vi "Data Sharing Framework Configuration Explorer.vi"(6 "menu options":cluster{"open":bool, "save":bool, "view":bool}={"open"=TRUE, "save"=FALSE, "view"=FALSE}, 8 "error in (no error)":errorcluster, 11 "Path in":path) -> (0 "error out":errorcluster, 3 "Path out":path)   [LabVIEW 2017]
uses:
  Main VI/Application Data.ctl
  VeriStand/Data Sharing Custom Device/Source/DSF Core.lvlibp/DSF Configuration API/Configuration Session.lvclass
  Main VI/View Mode.ctl
  Main VI/Load DSF Configuration File.vi
  Item Tree/Clear Tree.vi
  VeriStand/Data Sharing Custom Device/Source/DSF Core.lvlibp/DSF Configuration API/Public/Read DSF Version.vi
  Value Tree/variant to tree resources/View Variant in Tree.vi
  VeriStand/Data Sharing Custom Device/Source/DSF Core.lvlibp/DSF Configuration API/Private/File IO/Read Configuration Version.vi
  Item Tree/Get Item Type.vi
  Item Tree/Get Item Display Name.vi
  VeriStand/Data Sharing Custom Device/Source/DSF Core.lvlibp/DSF Configuration API/Public/Read Item.vi
  VeriStand/Data Sharing Custom Device/Source/DSF Core.lvlibp/DSF Configuration API/Public/Read Item/Read Group.vi
  VeriStand/Data Sharing Custom Device/Source/DSF Core.lvlibp/DSF Configuration API/Public/Read Item/Read Transfer.vi
  VeriStand/Data Sharing Custom Device/Source/DSF Core.lvlibp/DSF Configuration API/Public/Read Item/Read Channel.vi
  VeriStand/Data Sharing Custom Device/Source/DSF Core.lvlibp/DSF Configuration API/Public/Read Item/Read Settings.vi
  VeriStand/Data Sharing Custom Device/Source/DSF Core.lvlibp/DSF Configuration API/Public/Read Item/Read Plugin.vi
  DSF Configuration Utility.lvlib
panel:
  in  "Item Tree":string(tree)
  in  "Value Tree":string(tree)
  # "DSF Configuration Explorer"
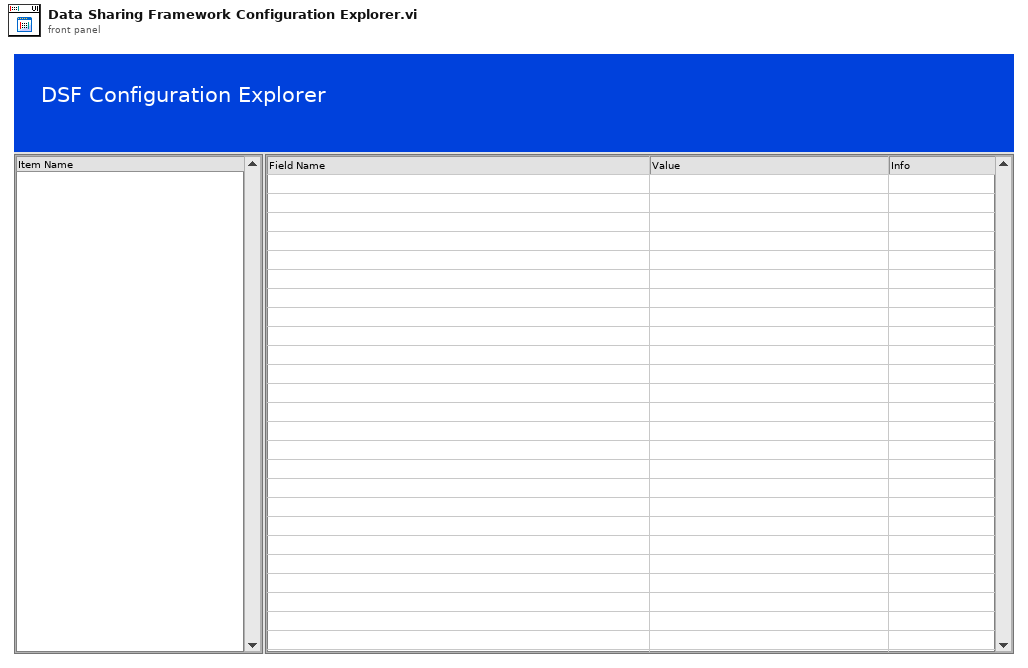
[diagram p1: front panel]
types:
  T1 = typedef "DSF Configuration Utility.lvlib/View Mode.ctl" = enum16{"Tree", "List"}
  T2 = typedef "DSF Configuration Utility.lvlib/Application Data.ctl" = cluster{"Item Tree Control":refnum<vi>, "Value Tree Control":refnum<vi>, "DSF Refnum":refnum<class "Configuration Session.lvclass">, "Top-Level VI":refnum<vi>, "View State":T1, "menu reference":refnum<k9>}
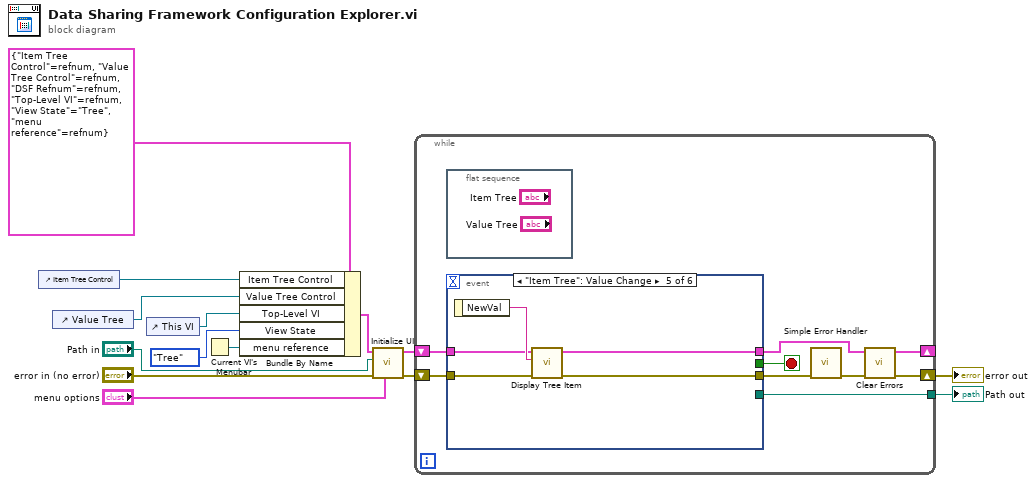
[diagram p0: block diagram]
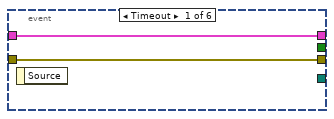
[diagram p2: hidden frame]
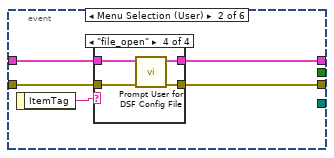
[diagram p3: hidden frame]
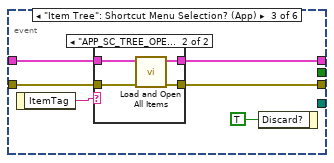
[diagram p7: hidden frame]
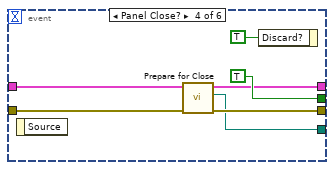
[diagram p9: hidden frame]
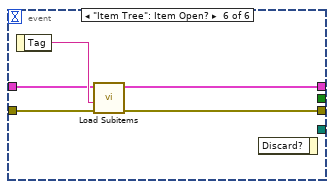
[diagram p10: hidden frame]
diagram:
  n1 = control-ref of="Item Tree Control"() -> (w2:refnum<vi>)
  n2 = control-ref of="Value Tree"() -> (w1:refnum<vi>)
  n3 = control-ref of="This VI"() -> (w11:refnum<vi>)
  n4 = Current VI's Menubar() -> (w6:refnum<k9>)
  n5 = Bundle By Name(cluster=T2 {"Item Tree Control"=refnum, "Value Tree Control"=refnum, "DSF Refnum"=refnum, "Top-Level VI"=refnum, "View State"=enum."Tree", "menu reference"=refnum}, "Item Tree Control"=w2, "Value Tree Control"=w1, "Top-Level VI"=w11, "View State"=View_Mode."Tree", "menu reference"=w6) -> (w4:T2)
  n6 = call "Initialize UI.vi"("menu options"="menu options", "error in (no error)"="error in (no error)", "Path"="Path in", "Application Data in"=w4) -> ("error out"=w14:errorcluster, "Application Data out"=w10:T2)  [unwired: 6 in]
  n7 = while {
    shift-right: [w15] -> w7
    shift-left: w14 -> [w21]
    shift-right: [w17] -> _
    shift-left: w10 -> [w18]
    tunnel: [w16] -> w8
    stop <- w22 stop-if-true
    n8 = flat-sequence {
      frame #0 {
      }
    }
    n9 = event shown="[4] \"Item Tree\": Value Change" {
      selector: _ -> [_ _ _ _ _ _]
      dyn-events: _ -> [_ _ _ _ _ _]
      timeout: _ -> [_ _ _ _ _ _]
      tunnel: [_ _ _ TRUE _ _] -> w22
      tunnel: w21 -> [w24 w28 w42 w57 w63 w68]
      tunnel: [w24 w27 w43 w54 w61 w67] -> w19
      tunnel: w18 -> [w23 w26 w44 w55 w59 w65]
      tunnel: [w23 w25 w40 w53 w60 w64] -> w17
      tunnel: [_ _ _ w52 _ _] -> w16
      event Timeout {
        n10 = event-data() -> ()  [unwired: 1 in, 1 out]
      }
      event Menu Selection (User) {
        n11 = event-data() -> ("ItemTag"=w29:string)  [unwired: 1 in]
        n12 = case shown="\"file_open\"" w29 {
          tunnel: [w30 w32 w34 w38] -> w25
          tunnel: [w31 w33 w35 w37] -> w27
          tunnel: w28 -> [w31 w33 w35 w39]
          tunnel: w26 -> [w30 w32 w34 w36]
          frame "view_tree" {
          }
          frame "view_list" {
          }
          frame Default {
          }
          frame "file_open" {
            n13 = call "Prompt User for DSF Config File.vi"("error in (no error)"=w39, "Application Data in"=w36) -> ("error out"=w37:errorcluster, "Application Data out"=w38:T2)  [unwired: 8 in]
          }
        }
      }
      event "Item Tree": Shortcut Menu Selection? (App) {
        n14 = event-data() -> ("ItemTag"=w45:string)  [unwired: 1 in]
        n15 = case shown="\"APP_SC_TREE_OPEN_ALL_ITEMS\"" w45 {
          tunnel: w44 -> [w46 w51]
          tunnel: [w47 w49] -> w43
          tunnel: w42 -> [w47 w50]
          tunnel: [w46 w48] -> w40
          frame Default {
          }
          frame "APP_SC_TREE_OPEN_ALL_ITEMS" {
            n16 = call "Load and Open All Items.vi"("error in (no error)"=w50, "Application Data in"=w51) -> ("error out"=w49:errorcluster, "Application Data out"=w48:T2)  [unwired: 8 in]
          }
        }
        n17 = event-data("Discard?"=TRUE) -> ()  [unwired: 1 in, 1 out]
      }
      event Panel Close? {
        n18 = event-data() -> ()  [unwired: 1 in, 1 out]
        n19 = call "Prepare for Close.vi"("error in (no error)"=w57, "Application Data in"=w55) -> ("error out"=w54:errorcluster, "file path"=w52:path, "Application Data out"=w53:T2)  [unwired: 7 in]
        n20 = event-data("Discard?"=TRUE) -> ()  [unwired: 1 in, 1 out]
      }
      event "Item Tree": Value Change {
        n21 = event-data() -> ("NewVal"=w62:string)  [unwired: 1 in]
        n22 = call "Display Tree Item.vi"("error in (no error)"=w63, "Tag"=w62, "Application Data in"=w59) -> ("error out"=w61:errorcluster, "Application Data out"=w60:T2)  [unwired: 7 in]
      }
      event "Item Tree": Item Open? {
        n23 = event-data() -> ("Tag"=w66:string)  [unwired: 1 in]
        n24 = call "Load Subitems.vi"("error in (no error)"=w68, "Tag"=w66, "Application Data in"=w65) -> ("error out"=w67:errorcluster, "Application Data out"=w64:T2)  [unwired: 6 in, 1 out]
        n25 = event-data() -> ()  [unwired: 2 in, 1 out]
      }
    }
    n26 = call <vilib>:"Simple Error Handler.vi"("error in (no error)"=w19) -> ("error out"=w20:errorcluster)  [unwired: 4 in, 4 out]
    n27 = call <vilib>:"Clear Errors.vi"("error in (no error)"=w20) -> ("error out"=w15:errorcluster)  [unwired: 5 in, 1 out]
  }
  "Path out" <- w8
  "error out" <- w7
